vi "AbsoluteRetract.vi"(8 "Z End":dbl=38.0, 9 "Z Start height":dbl, 10 "Distance To Retract / um":dbl=-1.0) -> (2 "Distance To Retract / um 2":dbl=-1.0)   [LabVIEW 2023]
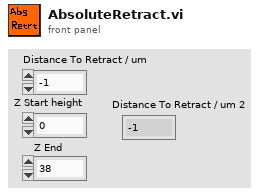
[diagram p1: front panel]
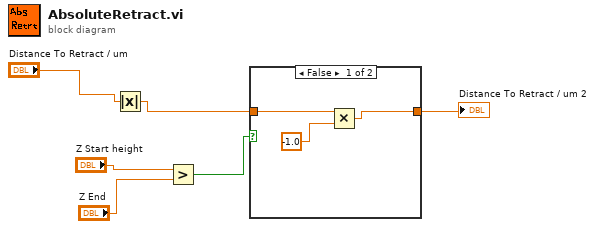
[diagram p0: block diagram]
diagram:
  n1 = Absolute Value(x="Distance To Retract / um") -> (abs(x)=w1:dbl)
  n2 = Greater?(x="Z Start height", y="Z End") -> (0:w4:bool)
  n3 = case shown="False" w4 {
    tunnel: [w7 w10] -> w3
    tunnel: w1 -> [w9 w10]
    frame False {
      n4 = Multiply(x=w9, y=-1.0) -> (x*y=w7:dbl)
    }
    frame True {
    }
  }
  "Distance To Retract / um 2" <- w3
